vi "Main.vi"() -> ()   [LabVIEW 2020]
doc: "Machine d'état première partie"
uses:
  Controller/Ctrl_enum_state.ctl
  Controller/Ctrl_Local.ctl
panel:
  in  "Btn_Arrêter":bool
  out "Led_Display":bool
  out "Str_Display":string
  in  "BTN_etat3":bool
  in  "BTN_etat2":bool
  in  "BTN_etat1":bool
  out "error out":errorcluster caption="sortie d'erreur"
  in  "error in":errorcluster caption="entrée d'erreur"
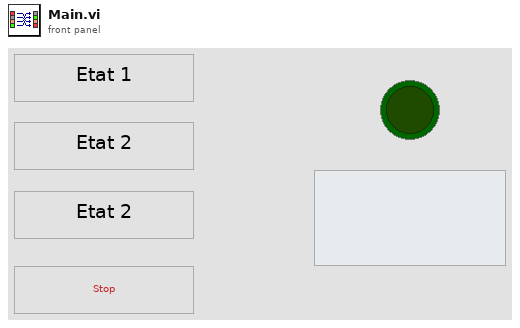
[diagram p1: front panel]
types:
  T1 = typedef "Ctrl_enum_state.ctl" = enum16{"Idle", "Init", "Display", "Etat 1", "Etat 2", "Etat 3", "Exit"}
  T2 = typedef "Ctrl_Local.ctl" = cluster{"Led_Display":bool, "Str_Display":string}
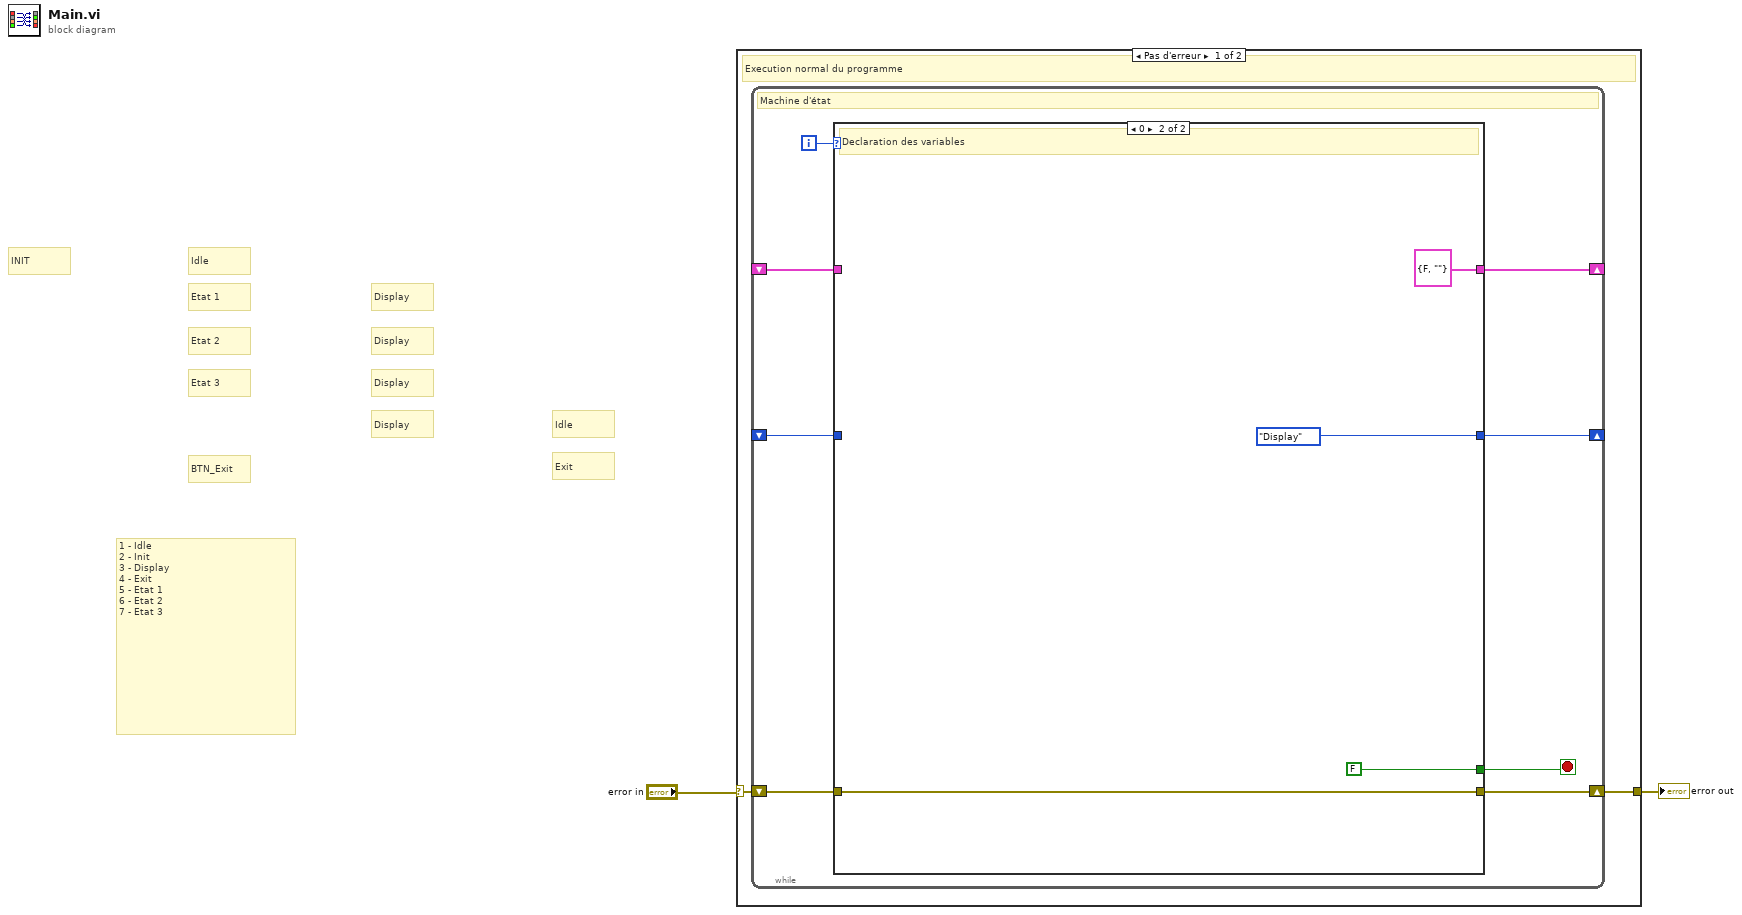
[diagram p0: block diagram]
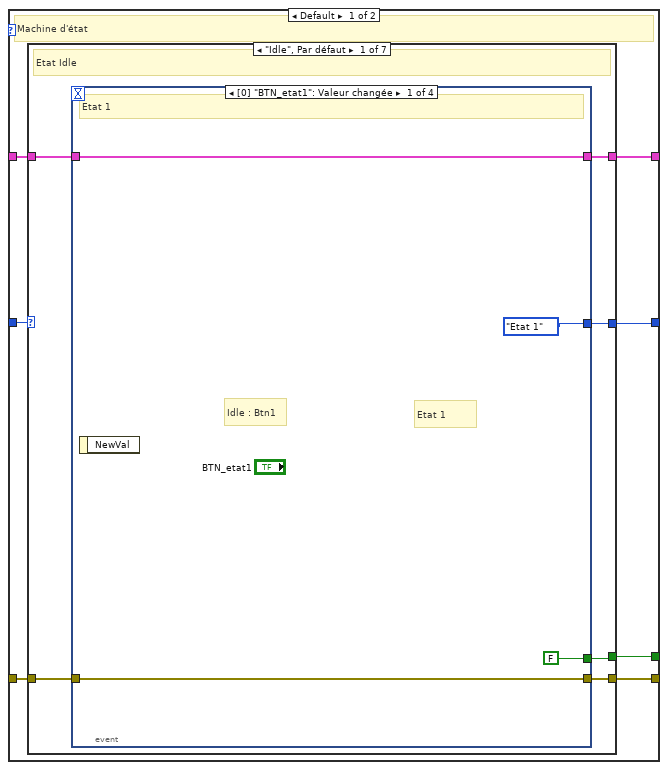
[diagram p2: hidden frame]
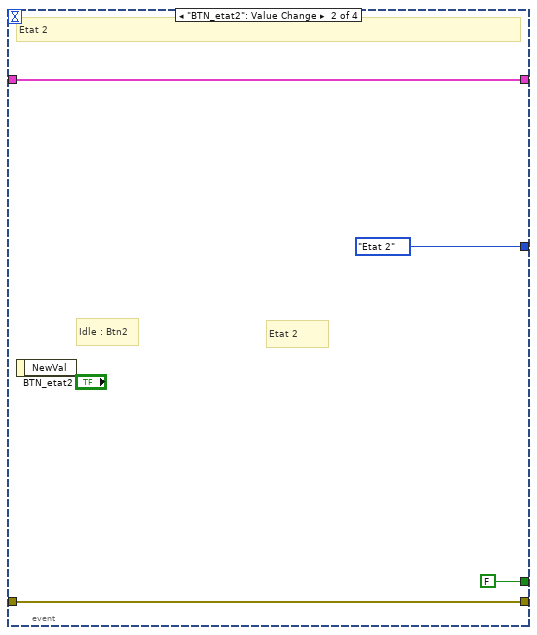
[diagram p3: hidden frame]
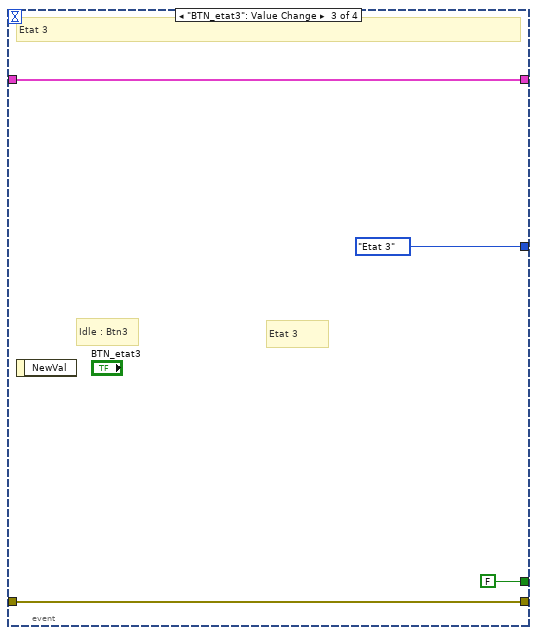
[diagram p4: hidden frame]
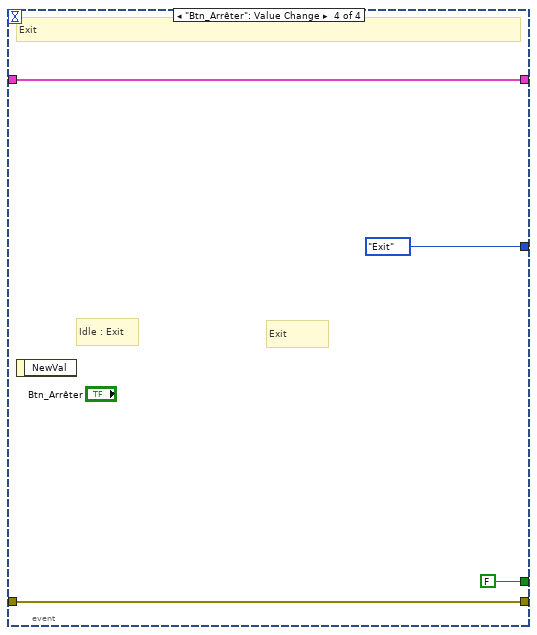
[diagram p5: hidden frame]
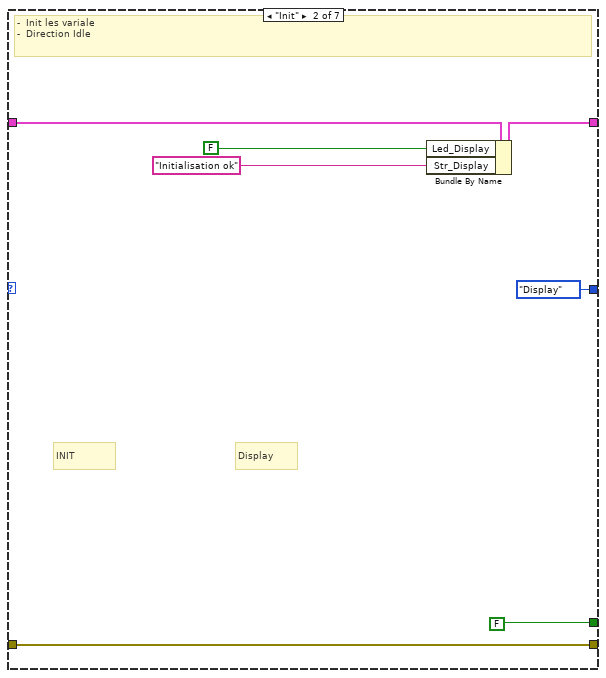
[diagram p6: hidden frame]
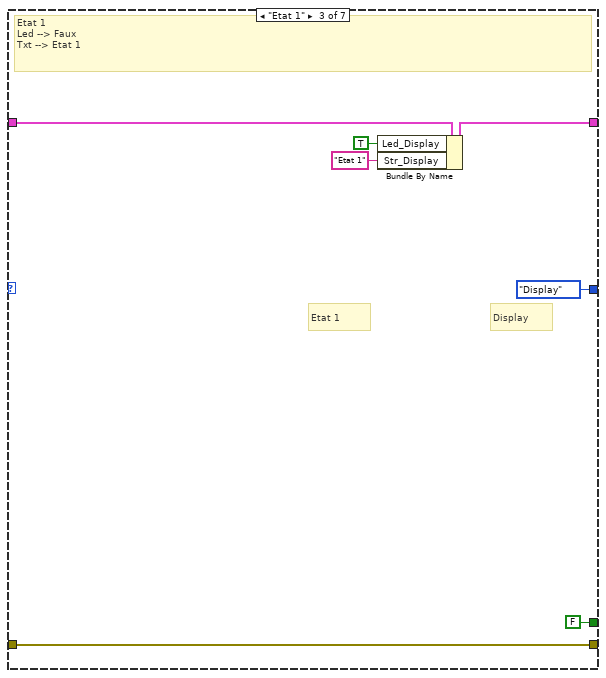
[diagram p7: hidden frame]
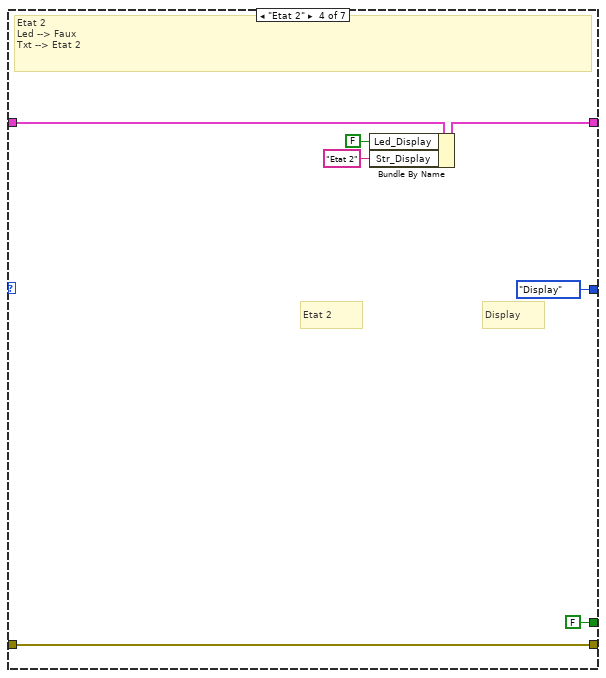
[diagram p8: hidden frame]
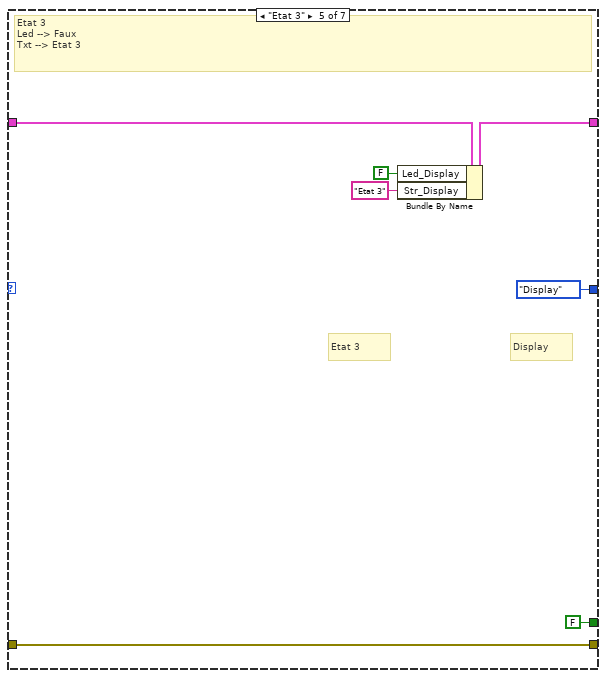
[diagram p9: hidden frame]
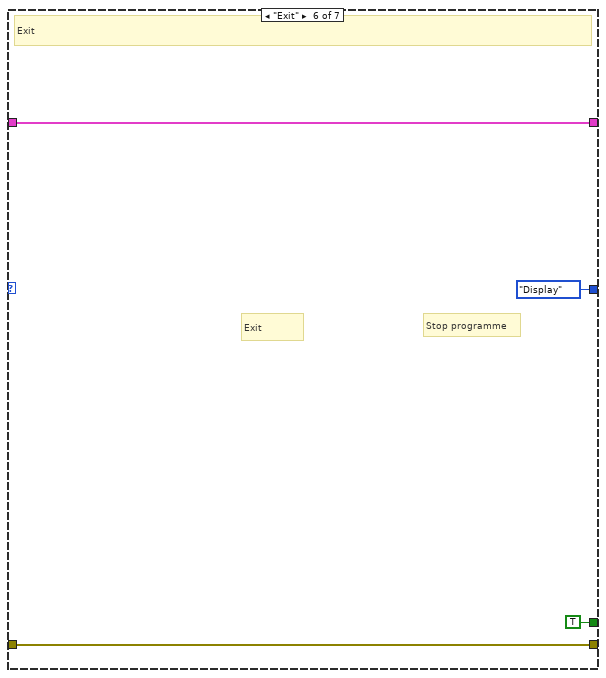
[diagram p10: hidden frame]
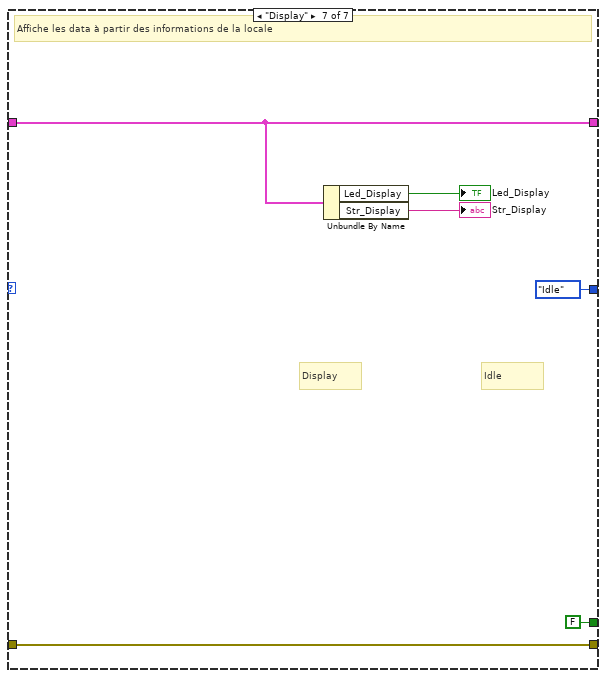
[diagram p11: hidden frame]
diagram:
  # "Exit"
  # "BTN_Exit"
  # "Idle"
  # "INIT"
  # "Display"
  # "Etat 1"
  # "Display"
  # "Etat 2"
  # "Display"
  # "Etat 3"
  # "Idle"
  # "Display"
  # "1 - Idle\n2 - Init\n3 - Display\n4 - Exit\n5 - Etat 1\n6 - Etat 2\n7 - Etat 3"
  n1 = case shown="Pas d'erreur" "error in" {
    selector: "error in" -> [w4 w84]
    tunnel: [w3 w84] -> w1
    frame No Error {
      # "Execution normal du programme"
      n2 = while {
        shift-right: [w11] -> w3
        shift-left: w4 -> [w12]
        shift-right: [w8] -> _
        shift-left: _ -> [w7]
        shift-right: [w5] -> _
        shift-left: _ -> [w6]
        i -> [w10]
        stop <- w9 stop-if-true
        # "Machine d'état"
        n3 = case shown="0" w10 {
          tunnel: w12 -> [w15 w83]
          tunnel: [w14 w83] -> w11
          tunnel: [w13 FALSE] -> w9
          tunnel: [w18 T2 {"Led_Display"=FALSE, "Str_Display"=""} ("Declaration_Local")] -> w8
          tunnel: w7 -> [w19 _]
          tunnel: w6 -> [w17 _]
          tunnel: [w16 Ctrl_enum_state."Display"] -> w5
          frame Default {
            # "Machine d'état"
            n4 = case shown="\"Idle\", Par défaut" w17 {
              tunnel: w19 -> [w25 w48 w55 w62 w69 w70 w79]
              tunnel: [w24 w47 w52 w59 w66 w70 w79] -> w18
              tunnel: [w20 Ctrl_enum_state."Display" Ctrl_enum_state."Display" Ctrl_enum_state."Display" Ctrl_enum_state."Display" Ctrl_enum_state."Display" Ctrl_enum_state."Idle"] -> w16
              tunnel: w15 -> [w23 w44 w54 w61 w68 w73 w76]
              tunnel: [w22 w44 w54 w61 w68 w73 w76] -> w14
              tunnel: [w21 FALSE FALSE FALSE FALSE TRUE FALSE] -> w13
              frame "Idle", Default {
                # "Etat Idle"
                n5 = event shown="[0] \"BTN_etat1\": Valeur changée" {
                  selector: _ -> [_ _ _ _]
                  dyn-events: _ -> [_ _ _ _]
                  timeout: _ -> [_ _ _ _]
                  tunnel: w25 -> [w27 w31 w35 w39]
                  tunnel: [w27 w31 w35 w39] -> w24
                  tunnel: w23 -> [w29 w33 w37 w41]
                  tunnel: [w29 w33 w37 w41] -> w22
                  tunnel: [FALSE FALSE FALSE FALSE] -> w21
                  tunnel: [Ctrl_enum_state."Etat 1" Ctrl_enum_state."Etat 2" Ctrl_enum_state."Etat 3" Ctrl_enum_state."Exit"] -> w20
                  event "BTN_etat1": Value Change {
                    # "Etat 1"
                    # "Idle : Btn1"
                    # "Etat 1"
                    n6 = event-data() -> ()  [unwired: 1 in, 1 out]
                  }
                  event "BTN_etat2": Value Change {
                    # "Etat 2"
                    # "Idle : Btn2"
                    # "Etat 2"
                    n7 = event-data() -> ()  [unwired: 1 in, 1 out]
                  }
                  event "BTN_etat3": Value Change {
                    # "Etat 3"
                    # "Idle : Btn3"
                    # "Etat 3"
                    n8 = event-data() -> ()  [unwired: 1 in, 1 out]
                  }
                  event "Btn_Arrêter": Value Change {
                    # "Exit"
                    # "Idle : Exit"
                    # "Exit"
                    n9 = event-data() -> ()  [unwired: 1 in, 1 out]
                  }
                }
              }
              frame "Init" {
                # "Display"
                # "INIT"
                # "-  Init les variale \n-  Direction Idle"
                n10 = Bundle By Name(cluster=w48, "Led_Display"=FALSE, "Str_Display"="Initialisation ok") -> (w47:T2)
              }
              frame "Etat 1" {
                # "Display"
                # "Etat 1"
                # "Etat 1\nLed --> Faux\nTxt --> Etat 1"
                n11 = Bundle By Name(cluster=w55, "Led_Display"=TRUE, "Str_Display"="Etat 1") -> (w52:T2)
              }
              frame "Etat 2" {
                # "Display"
                # "Etat 2"
                # "Etat 2\nLed --> Faux\nTxt --> Etat 2"
                n12 = Bundle By Name(cluster=w62, "Led_Display"=FALSE, "Str_Display"="Etat 2") -> (w59:T2)
              }
              frame "Etat 3" {
                # "Display"
                # "Etat 3"
                # "Etat 3\nLed --> Faux\nTxt --> Etat 3"
                n13 = Bundle By Name(cluster=w69, "Led_Display"=FALSE, "Str_Display"="Etat 3") -> (w66:T2)
              }
              frame "Exit" {
                # "Stop programme"
                # "Exit"
                # "Exit"
              }
              frame "Display" {
                # "Idle"
                # "Display"
                # "Affiche les data à partir des informations de la locale"
                n14 = Unbundle By Name(w79) -> ("Led_Display"=→"Led_Display":bool, "Str_Display"=→"Str_Display":string)
              }
            }
          }
          frame 0 {
            # "Declaration des variables"
          }
        }
      }
    }
    frame Error {
      # "Erreur on laisse passer le flux"
    }
  }
  "error out" <- w1
